vi "Start Server.vi"(8 "error in (no error)":errorcluster, 11 "gRPC Server in":refnum<class "HVC2.lvclass">) -> (0 "error out":errorcluster, 3 "gRPC Server out":refnum<class "HVC2.lvclass">)   [LabVIEW 2019, in "HVC2.lvlib" / "HVC2.lvclass"]
uses:
  HVC2.lvclass
  HVC2.lvclass/HVC2.ctl
  gRPC lvSupport/gprc-lvsupport.lvlib
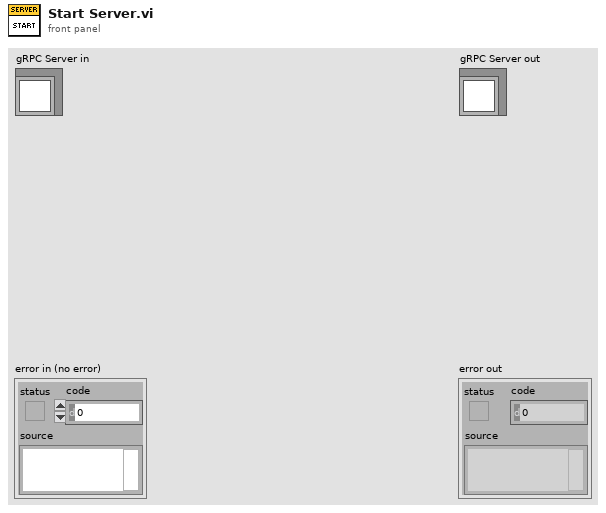
[diagram p1: front panel]
types:
  T1 = typedef "HVC2.lvlib/gprc-lvsupport.lvlib/grpcId.ctl" = u64
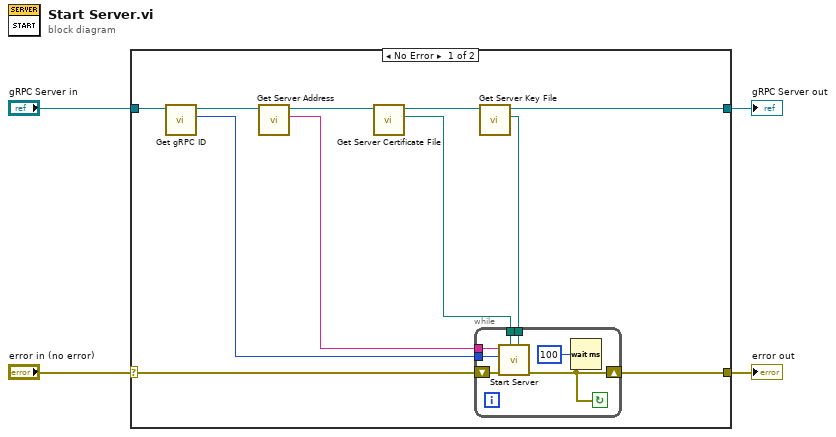
[diagram p0: block diagram]
diagram:
  n1 = case shown="No Error" "error in (no error)" {
    selector: "error in (no error)" -> [w15 w24]
    tunnel: [w5 w24] -> w3
    tunnel: [w6 w23] -> w1
    tunnel: "gRPC Server in" -> [w13 w23]
    frame No Error {
      n2 = call "Get gRPC ID.vi"("OOP Server in"=w13) -> ("gRPC ID"=w11:T1, "OOP Server out"=w12:refnum<class "HVC2.lvclass">)  [unwired: 9 in]
      n3 = call "Get Server Address.vi"("OOP Server in"=w12) -> ("Server Address"=w14:string, "OOP Server out"=w10:refnum<class "HVC2.lvclass">)  [unwired: 9 in]
      n4 = call "Get Server Certificate File.vi"("OOP Server in"=w10) -> ("Server Certificate File (.crt)"=w9:path, "OOP Server out"=w8:refnum<class "HVC2.lvclass">)  [unwired: 9 in]
      n5 = call "Get Server Key File.vi"("OOP Server in"=w8) -> ("Server Key File (.key)"=w7:path, "OOP Server out"=w6:refnum<class "HVC2.lvclass">)  [unwired: 9 in]
      n6 = while {
        tunnel: w14 -> [w21]
        tunnel: w11 -> [w20]
        tunnel: w9 -> [w19]
        tunnel: w7 -> [w18]
        shift-right: [w16] -> w5
        shift-left: w15 -> [w22]
        stop <- w16 continue-if-true
        n7 = call "Start Server.vi"("Server Key File (.key)"=w18, "Server Certificate File (.crt)"=w19, "error in (no error)"=w22, "gRPCid"=w20, "Server Address"=w21) -> ("error out"=w16:errorcluster)  [unwired: 6 in]
        n8 = Wait (ms)(milliseconds to wait=u32 100) -> ()  [unwired: 1 out]
      }
    }
    frame Error {
    }
  }
  "error out" <- w3
  "gRPC Server out" <- w1
